vi "configure.vi"(8 "error in (no error)":errorcluster, 11 "StageMG100204SutterMP285 in":refnum<class "StageMG100204SutterMP285.lvclass">=refnum) -> (0 "error out":errorcluster, 3 "StageMG100204SutterMP285 out":refnum<class "StageMG100204SutterMP285.lvclass">)   [LabVIEW 2010, in "StageMG100204SutterMP285.lvclass"]
doc: "The dynamic dispatch version of this VI loads and displays the configuration file associated with the plug-in object. The user modify and save the configuration data."
uses:
  StageMG100204SutterMP285.lvclass
panel:
  in  "cancel button":bool
  in  "save button":bool
  in  "LoRes Speed (fast)":dbl=750.0
  in  "HiRes Speed (slow)":dbl=100.0
  in  "serial port name":dbl
  # "Configure StageMG100204SutterMP285"
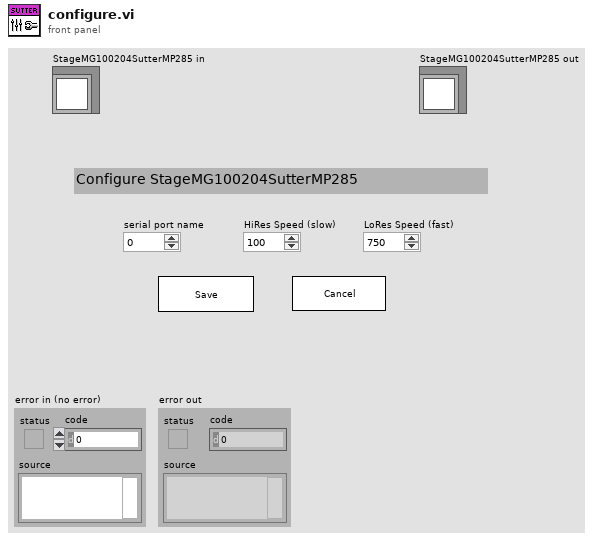
[diagram p1: front panel]
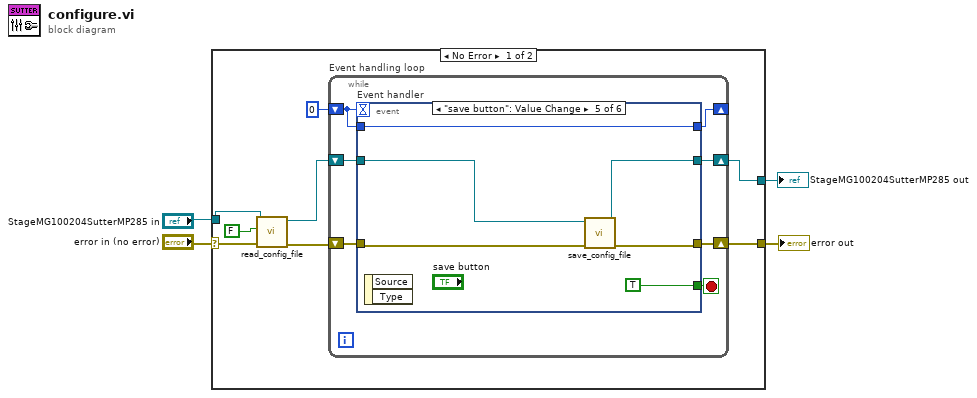
[diagram p0: block diagram]
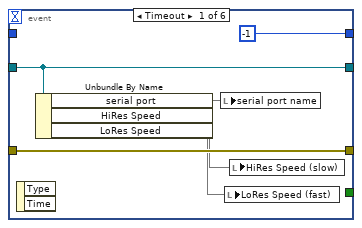
[diagram p2: hidden frame]
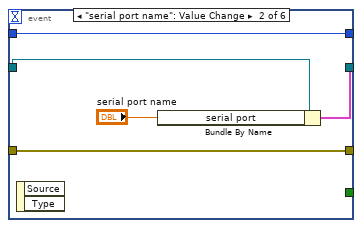
[diagram p3: hidden frame]
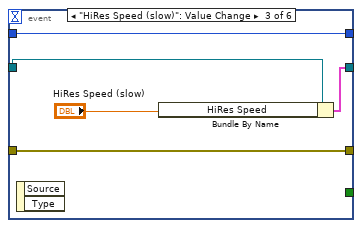
[diagram p4: hidden frame]
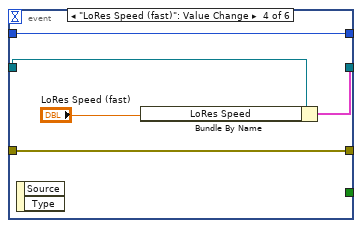
[diagram p5: hidden frame]
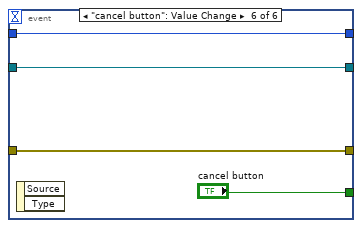
[diagram p6: hidden frame]
diagram:
  n1 = case shown="No Error" "error in (no error)" {
    selector: "error in (no error)" -> [w8 w52]
    tunnel: [w12 w52] -> w3
    tunnel: "StageMG100204SutterMP285 in" -> [w7 w51]
    tunnel: [w11 w51] -> w1
    frame No Error {
      n2 = call-dynamic "read_config_file.vi"("error in (no error)"=w8, "force load?"=FALSE, "StageMG100204SutterMP285 in"=w7) -> ("error out"=w9:errorcluster, "StageMG100204SutterMP285 out"=w6:refnum<class "StageMG100204SutterMP285.lvclass">)  [unwired: 7 in]
      n3 = while "Event handling loop" {
        shift-right: [w18] -> w12
        shift-left: w9 -> [w19]
        shift-right: [w17] -> w11
        shift-left: w6 -> [w13]
        shift-right: [w15] -> _
        shift-left: 0 -> [w16]
        stop <- w14 stop-if-true
        n4 = event "Event handler" shown="[4] \"save button\": Value Change" {
          selector: _ -> [_ _ _ _ _ _]
          dyn-events: _ -> [_ _ _ _ _ _]
          timeout: w16 -> [_ _ _ _ _ _]
          tunnel: w19 -> [w25 w30 w35 w40 w44 w50]
          tunnel: [w25 w30 w35 w40 w43 w50] -> w18
          tunnel: [w23 w27 w32 w37 w42 w47] -> w17
          tunnel: [-1 w29 w34 w39 w46 w49] -> w15
          tunnel: w16 -> [_ w29 w34 w39 w46 w49]
          tunnel: [_ _ _ _ TRUE "cancel button"] -> w14
          tunnel: w13 -> [w23 w28 w33 w38 w41 w47]
          event Timeout {
            n5 = event-data() -> ()  [unwired: 3 out]
            n6 = Unbundle By Name(w23) -> ("serial port"=w22, "HiRes Speed"=w21, "LoRes Speed"=w20)
            n7 = local write "serial port name"(w22) -> ()
            n8 = local write "LoRes Speed (fast)"(w20) -> ()
            n9 = local write "HiRes Speed (slow)"(w21) -> ()
          }
          event "serial port name": Value Change {
            n10 = event-data() -> ()  [unwired: 3 out]
            n11 = Bundle By Name(cluster=w28, "serial port"="serial port name") -> (w27:cluster{})
          }
          event "HiRes Speed (slow)": Value Change {
            n12 = event-data() -> ()  [unwired: 3 out]
            n13 = Bundle By Name(cluster=w33, "HiRes Speed"="HiRes Speed (slow)") -> (w32:cluster{})
          }
          event "LoRes Speed (fast)": Value Change {
            n14 = event-data() -> ()  [unwired: 3 out]
            n15 = Bundle By Name(cluster=w38, "LoRes Speed"="LoRes Speed (fast)") -> (w37:cluster{})
          }
          event "save button": Value Change {
            n16 = event-data() -> ()  [unwired: 3 out]
            n17 = call-dynamic "save_config_file.vi"("error in (no error)"=w44, "StageMG100204SutterMP285 in"=w41) -> ("error out"=w43:errorcluster, "StageMG100204SutterMP285 out"=w42:refnum<class "StageMG100204SutterMP285.lvclass">)  [unwired: 8 in]
          }
          event "cancel button": Value Change {
            n18 = event-data() -> ()  [unwired: 3 out]
          }
        }
      }
    }
    frame Error {
    }
  }
  "error out" <- w3
  "StageMG100204SutterMP285 out" <- w1
